vi "Calculate Offspring.vi"(7 "Days":i32, 11 "Age":i8) -> (2 "Population":i8[](array[numeric]), 3 "Offspring":dbl format="%#_6f")   [LabVIEW 2021]
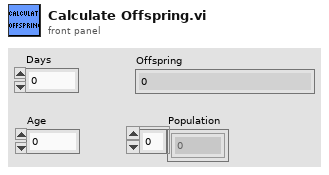
[diagram p1: front panel]
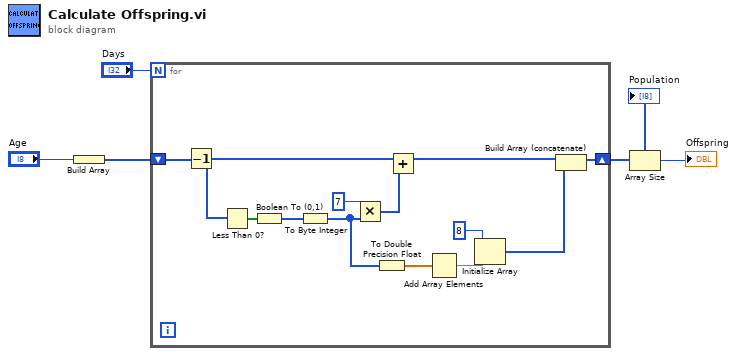
[diagram p0: block diagram]
diagram:
  n1 = Build Array("Age") -> (w4:i8[])
  n2 = for {
    N: "Days" -> [_]
    shift-right: [w15] -> w2
    shift-left: w4 -> [w18]
    n3 = Decrement(x=w18) -> (x-1=w6:i8[])
    n4 = Less Than 0?(x=w6) -> (x < 0?=w14:bool[])
    n5 = Boolean To (0,1)(Boolean=w14) -> (0, 1=w10:i16[])
    n6 = To Byte Integer(number=w10) -> (8bit integer=w9:i8[])
    n7 = Multiply(x=i8 7, y=w9) -> (x*y=w11:i8[])
    n8 = To Double Precision Float(number=w9) -> (double precision float=w8:dbl[])
    n9 = Add(x=w6, y=w11) -> (x+y=w13:i8[])
    n10 = Add Array Elements(numeric array=w8) -> (sum=w7:dbl)
    n11 = Initialize Array(i8 8, w7) -> (w16:i8[])
    n12 = Build Array (concatenate)(w13, w16) -> (w15:i8[])
  }
  "Population" <- w2
  n13 = Array Size(array=w2) -> (size(s)=→"Offspring":i32)
